vi "Category Manager GUI.vi"(8 "error in (no error)":errorcluster, 11 "Database.lvclass":refnum<class "Account History.lvclass">) -> (0 "error out":errorcluster, 3 "Database.lvclass":refnum<class "Account History.lvclass">)   [LabVIEW 2018]
uses:
  support/classes/database/Account History.lvclass
  <vilib>/Utility/miscctls.llb/LVRowAndColumnTypeDef.ctl
  support/classes/CategoryList/CategoryList.lvclass
panel:
  in  "Clear Amount":bool
  in  "Edit Amount":bool
  in  "Rename":bool
  in  "Delete":bool
  in  "Add":bool
  in  "Category Name":string
  in  "Category Table":i32(listbox)
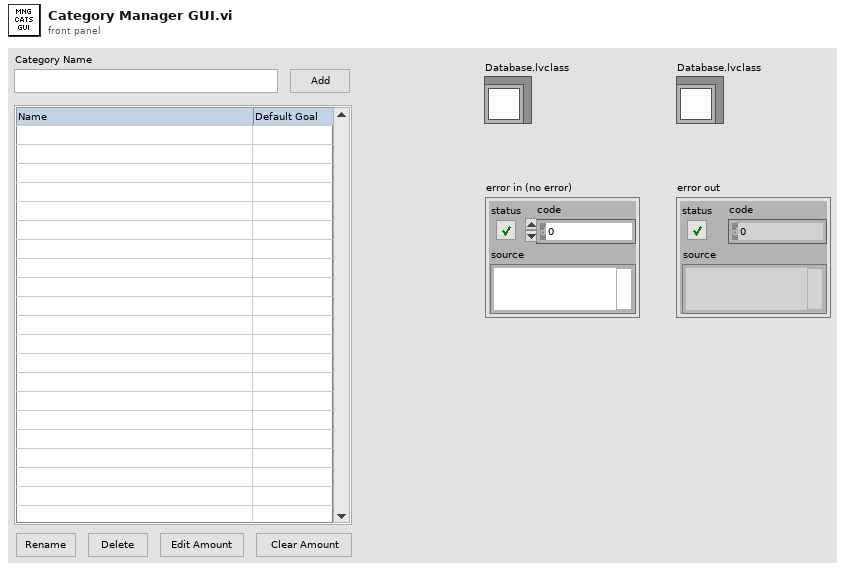
[diagram p1: front panel]
types:
  T1 = typedef "LVRowAndColumnTypeDef.ctl" = cluster{"Row":i32, "Column":i32}
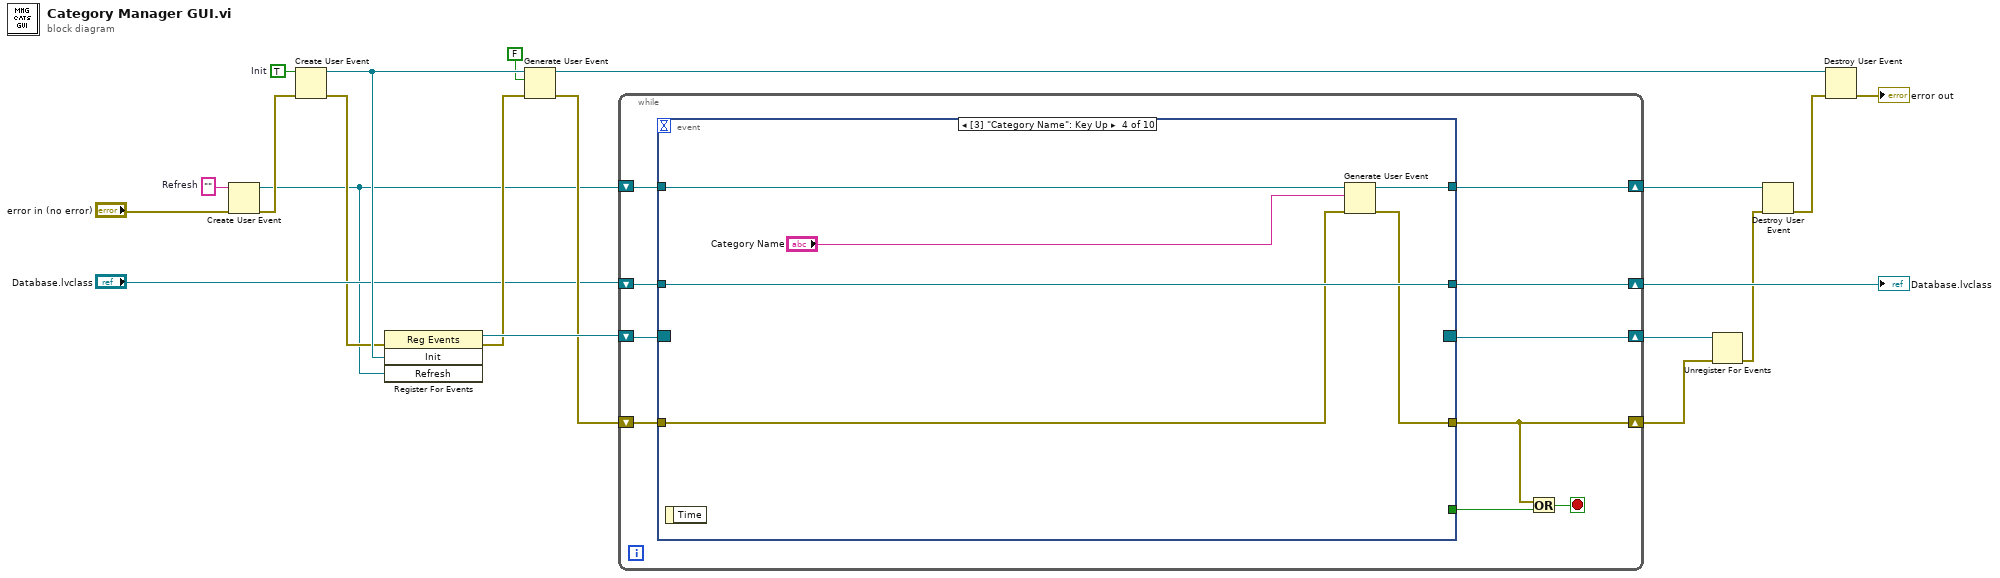
[diagram p0: block diagram]
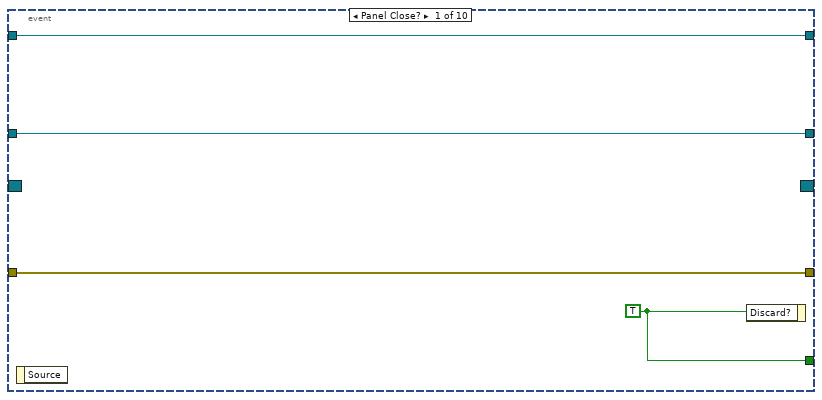
[diagram p2: hidden frame]
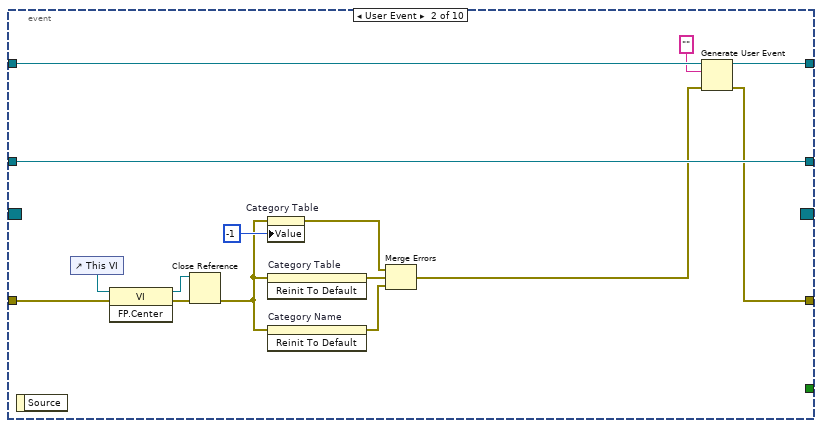
[diagram p3: hidden frame]
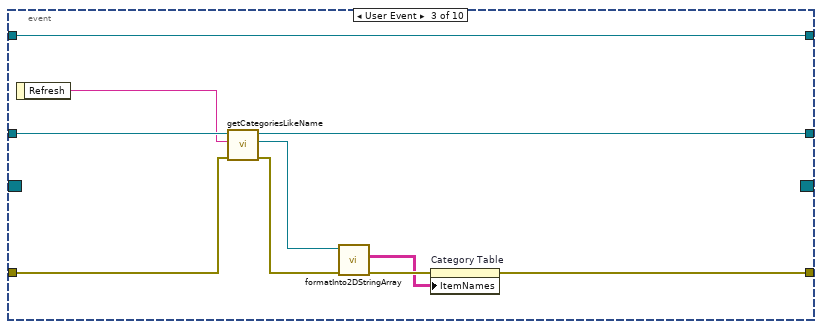
[diagram p4: hidden frame]
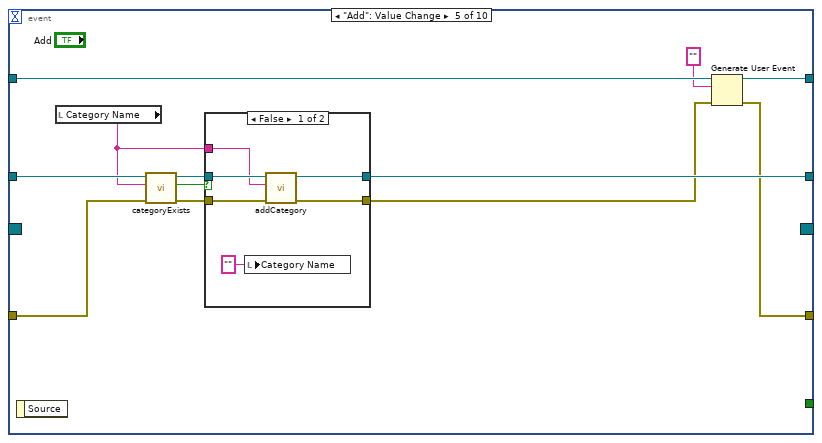
[diagram p5: hidden frame]
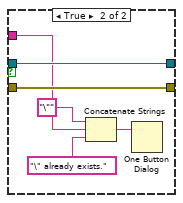
[diagram p6: hidden frame]
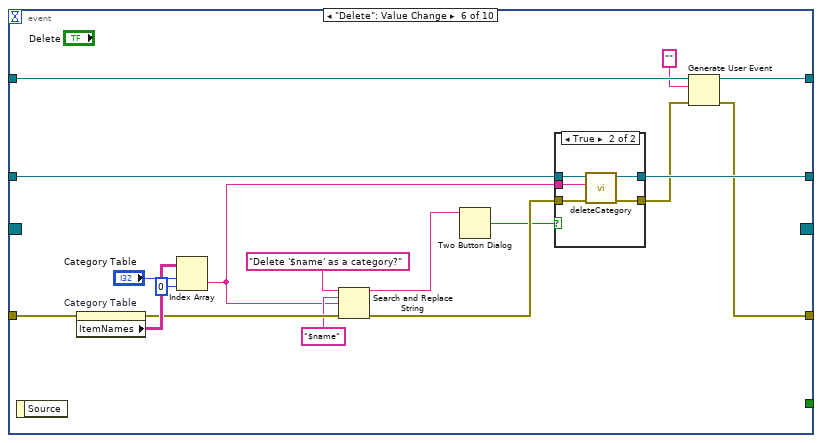
[diagram p7: hidden frame]
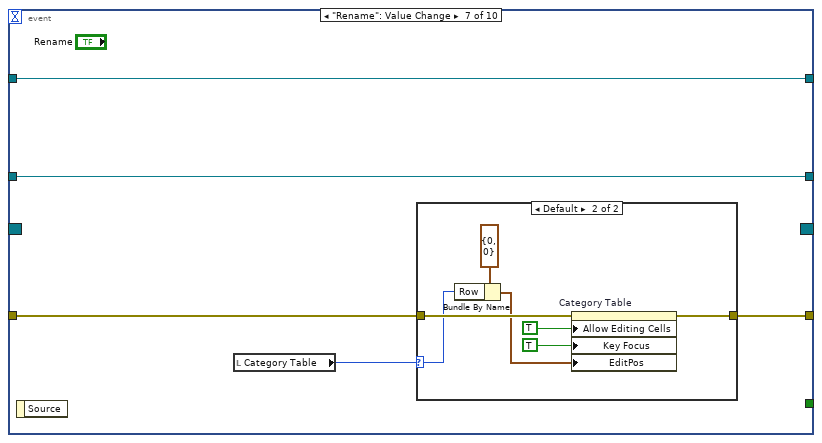
[diagram p9: hidden frame]
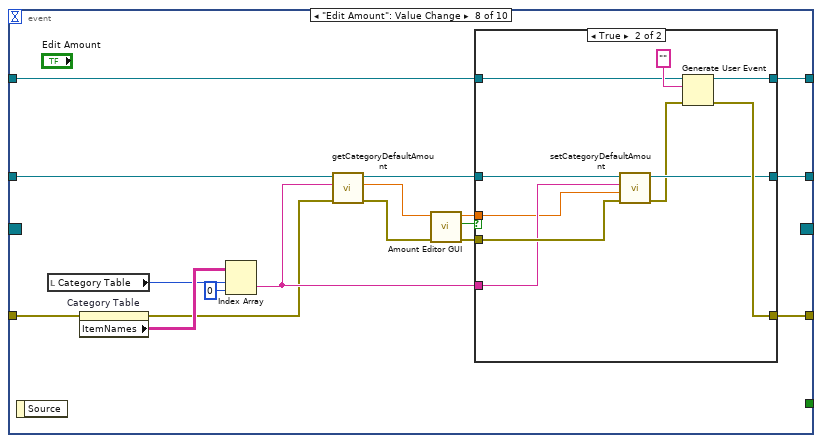
[diagram p11: hidden frame]
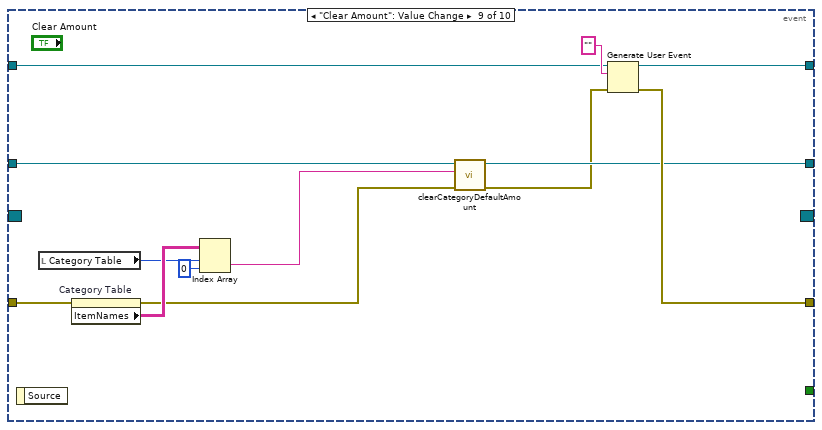
[diagram p13: hidden frame]
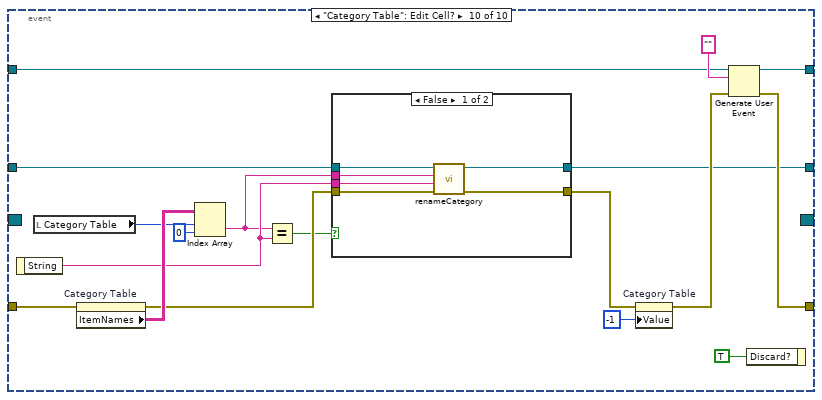
[diagram p14: hidden frame]
diagram:
  w1 = ""  # Refresh
  w20 = TRUE  # Init
  n1 = Create User Event(user event datatype=w1, error in="error in (no error)") -> (user event=w2:refnum<user-event>, error out=w4:errorcluster)
  n2 = Create User Event(user event datatype=w20, error in=w4) -> (user event=w18:refnum<user-event>, error out=w12:errorcluster)
  n3 = register-events(error in=w12, w18, w2) -> (reference out=w19:refnum<event-registration>, error out=w17:errorcluster)  [unwired: 1 in]
  n4 = Generate User Event(user event=w18, event data cluster=FALSE ("event data"), error in=w17) -> (user event out=w11:refnum<user-event>, error out=w16:errorcluster)  [unwired: 1 in]
  n5 = while {
    shift-right: [w28] -> w9
    shift-left: w19 -> [w30]
    shift-right: [w27] -> w8
    shift-left: w16 -> [w29]
    shift-right: [w23] -> w13
    shift-left: "Database.lvclass" -> [w24]
    shift-right: [w21] -> w5
    shift-left: w2 -> [w22]
    stop <- w25 stop-if-true
    n6 = event shown="[3] \"Category Name\": Key Up" {
      selector: w30 -> [_ _ _ _ _ _ _ _ _ _]
      dyn-events: [_ _ _ _ _ _ _ _ _ _] -> w28
      timeout: _ -> [_ _ _ _ _ _ _ _ _ _]
      tunnel: [w34 _ _ _ _ _ _ _ _ _] -> w26
      tunnel: w29 -> [w33 w45 w56 w61 w72 w107 w119 w138 w167 w186]
      tunnel: [w33 w36 w55 w62 w68 w100 w118 w142 w163 w180] -> w27
      tunnel: w24 -> [w32 w40 w58 w65 w74 w97 w116 w133 w162 w178]
      tunnel: [w32 w40 w57 w65 w71 w104 w116 w134 w161 w177] -> w23
      tunnel: w22 -> [w31 w39 w59 w64 w69 w102 w115 w143 w165 w181]
      tunnel: [w31 w38 w59 w63 w70 w103 w115 w144 w164 w182] -> w21
      event Panel Close? {
        w34 = TRUE ("Discard?")
        n7 = event-data() -> ()  [unwired: 1 in, 1 out]
        n8 = event-data("Discard?"=w34) -> ()  [unwired: 1 in, 1 out]
      }
      event User Event {
        n9 = event-data() -> ()  [unwired: 1 in, 1 out]
        n10 = control-ref of="This VI"() -> (w46:refnum<vi>)
        n11 = invoke class="VI" method="FP.Center"(reference=w46, error in=w45) -> (reference out=w43:refnum<vi>, error out=w44:errorcluster)  [unwired: 1 in, 1 out]
        n12 = Close Reference(reference=w43, error in (no error)=w44) -> (error out=w42:errorcluster)
        n13 = property on="Category Table" class="MCListbox (strict)"(error in=w42, "Value"=-1 ("Category Table")) -> (error out=w41:errorcluster)  [unwired: 1 in, 1 out]
        n14 = invoke on="Category Table" class="MCListbox (strict)" method="Reinit To Default"(error in=w42) -> (error out=w48:errorcluster)  [unwired: 2 in, 2 out]
        n15 = invoke on="Category Name" class="Str" method="Reinit To Default"(error in=w42) -> (error out=w49:errorcluster)  [unwired: 2 in, 2 out]
        n16 = Merge Errors(w41, w48, w49) -> (w37:errorcluster)
        n17 = Generate User Event(user event=w39, event data cluster="" ("event data"), error in=w37) -> (user event out=w38:refnum<user-event>, error out=w36:errorcluster)  [unwired: 1 in]
      }
      event User Event {
        n18 = event-data() -> ("Refresh"=w54:string)  [unwired: 1 in]
        n19 = call "getCategoriesLikeName.vi"("error in (no error)"=w56, "Name filter"=w54, "Database in"=w58) -> ("error out"=w52:errorcluster, "CategoryList out"=w53:refnum<class "CategoryList.lvclass">, "Database out"=w57:refnum<class "Account History.lvclass">)  [unwired: 6 in]
        n20 = call "formatInto2DStringArray.vi"("error in (no error)"=w52, "CategoryList in"=w53) -> ("error out"=w51:errorcluster, "2D String Array"=w50:string[][])  [unwired: 7 in, 1 out]
        n21 = property on="Category Table" class="MCListbox (strict)"(error in=w51, "ItemNames"=w50) -> (error out=w55:errorcluster)  [unwired: 1 in, 1 out]
      }
      event "Category Name": Key Up {
        n22 = event-data() -> ()  [unwired: 1 in, 1 out]
        n23 = Generate User Event(user event=w64, event data cluster="Category Name", error in=w61) -> (user event out=w63:refnum<user-event>, error out=w62:errorcluster)  [unwired: 1 in]
      }
      event "Add": Value Change {
        n24 = event-data() -> ()  [unwired: 1 in, 1 out]
        n25 = local read "Category Name"() -> (w73:string)
        n26 = call "categoryExists.vi"("error in (no error)"=w72, "Category Name"=w73, "Account History in"=w74) -> ("error out"=w76:errorcluster, "Exist?"=w77:bool, "Account History out"=w75:refnum<class "Account History.lvclass">)  [unwired: 6 in]
        n27 = case shown="False" w77 {
          tunnel: w76 -> [w82 w88]
          tunnel: w75 -> [w83 w89]
          tunnel: [w81 w89] -> w71
          tunnel: [w80 w88] -> w67
          tunnel: w73 -> [w79 w86]
          frame False {
            n28 = local write "Category Name"("" ("Category Name")) -> ()
            n29 = call "addCategory.vi"("error in (no error)"=w82, "name"=w79, "Database in"=w83) -> ("error out"=w80:errorcluster, "Database out"=w81:refnum<class "Account History.lvclass">)  [unwired: 7 in]
          }
          frame True {
            n30 = Concatenate Strings("\"" ("string"), w86, "\" already exists." ("string")) -> (w85:string)
            n31 = One Button Dialog(message=w85) -> ()  [unwired: 1 in, 1 out]
          }
        }
        n32 = Generate User Event(user event=w69, event data cluster="" ("Category Name"), error in=w67) -> (user event out=w70:refnum<user-event>, error out=w68:errorcluster)  [unwired: 1 in]
      }
      event "Delete": Value Change {
        n33 = event-data() -> ()  [unwired: 1 in, 1 out]
        n34 = property on="Category Table" class="MCListbox (strict)"(error in=w107) -> (error out=w96:errorcluster, "ItemNames"=w106:string[][])  [unwired: 1 in, 1 out]
        n35 = Index Array(array=w106, index (row)="Category Table", index (col)=0 ("disabled index (col)")) -> (element=w92:string)
        n36 = Search and Replace String(input string="Delete '$name' as a category?", search string="$name", replace string=w92, error in=w96) -> (result string=w91:string, error out=w95:errorcluster)  [unwired: 4 in, 2 out]
        n37 = Two Button Dialog(message=w91) -> (T button?=w90:bool)  [unwired: 2 in]
        n38 = case shown="True" w90 {
          tunnel: [w109 w114] -> w104
          tunnel: [w108 w113] -> w101
          tunnel: w97 -> [w109 w112]
          tunnel: w95 -> [w108 w111]
          tunnel: w92 -> [_ w110]
          frame False {
          }
          frame True {
            n39 = call "deleteCategory.vi"("error in (no error)"=w111, "Category Name"=w110, "Database in"=w112) -> ("error out"=w113:errorcluster, "Database out"=w114:refnum<class "Account History.lvclass">)  [unwired: 7 in]
          }
        }
        n40 = Generate User Event(user event=w102, event data cluster="" ("event data"), error in=w101) -> (user event out=w103:refnum<user-event>, error out=w100:errorcluster)  [unwired: 1 in]
      }
      event "Rename": Value Change {
        n41 = event-data() -> ()  [unwired: 1 in, 1 out]
        n42 = local read "Category Table"() -> (w117:i32)
        n43 = case shown="Default" w117 {
          selector: w117 -> [_ w121]
          tunnel: w119 -> [w120 w127]
          tunnel: [w120 w125] -> w118
          frame ..-1 {
          }
          frame Default {
            n44 = Bundle By Name(cluster=T1 {"Row"=0, "Column"=0} ("Edit Position"), "Row"=w121) -> (w122:T1)
            n45 = property on="Category Table" class="MCListbox (strict)"(error in=w127, "Allow Editing Cells"=TRUE, "Key Focus"=TRUE, "EditPos"=w122) -> (error out=w125:errorcluster)  [unwired: 1 in, 1 out]
          }
        }
      }
      event "Edit Amount": Value Change {
        n46 = event-data() -> ()  [unwired: 1 in, 1 out]
        n47 = local read "Category Table"() -> (w140:i32)
        n48 = property on="Category Table" class="MCListbox (strict)"(error in=w138) -> (error out=w130:errorcluster, "ItemNames"=w141:string[][])  [unwired: 1 in, 1 out]
        n49 = Index Array(array=w141, index (row)=w140, index (col)=0 ("disabled index (col)")) -> (element=w131:string)
        n50 = call "getCategoryDefaultAmount.vi"("error in (no error)"=w130, "Name"=w131, "Account History in"=w133) -> ("error out"=w129:errorcluster, "Default Amount"=w128:dbl, "Account History out"=w132:refnum<class "Account History.lvclass">)  [unwired: 6 in]
        n51 = call "Amount Editor GUI.vi"("error in (no error)"=w129, "Input Amount"=w128) -> ("error out"=w135:errorcluster, "UserConfirm?"=w136:bool, "Output Amount"=w137:dbl)  [unwired: 7 in]
        n52 = case shown="True" w136 {
          tunnel: [w147 w156] -> w144
          tunnel: w143 -> [w147 w155]
          tunnel: [w145 w154] -> w142
          tunnel: w137 -> [_ w148]
          tunnel: w135 -> [w145 w150]
          tunnel: w132 -> [w146 w153]
          tunnel: [w146 w152] -> w134
          tunnel: w131 -> [_ w149]
          frame False {
          }
          frame True {
            n53 = call "setCategoryDefaultAmount.vi"("error in (no error)"=w150, "Default Amount"=w148, "Name"=w149, "Account History in"=w153) -> ("error out"=w151:errorcluster, "Account History out"=w152:refnum<class "Account History.lvclass">)  [unwired: 6 in]
            n54 = Generate User Event(user event=w155, event data cluster="" ("event data"), error in=w151) -> (user event out=w156:refnum<user-event>, error out=w154:errorcluster)  [unwired: 1 in]
          }
        }
      }
      event "Clear Amount": Value Change {
        n55 = event-data() -> ()  [unwired: 1 in, 1 out]
        n56 = local read "Category Table"() -> (w169:i32)
        n57 = property on="Category Table" class="MCListbox (strict)"(error in=w167) -> (error out=w159:errorcluster, "ItemNames"=w170:string[][])  [unwired: 1 in, 1 out]
        n58 = Index Array(array=w170, index (row)=w169, index (col)=0 ("disabled index (col)")) -> (element=w158:string)
        n59 = call "clearCategoryDefaultAmount.vi"("error in (no error)"=w159, "Name"=w158, "Account History in"=w162) -> ("error out"=w160:errorcluster, "Account History out"=w161:refnum<class "Account History.lvclass">)  [unwired: 7 in]
        n60 = Generate User Event(user event=w165, event data cluster="" ("event data"), error in=w160) -> (user event out=w164:refnum<user-event>, error out=w163:errorcluster)  [unwired: 1 in]
      }
      event "Category Table": Edit Cell? {
        n61 = event-data() -> ("String"=w174:string)  [unwired: 1 in]
        n62 = local read "Category Table"() -> (w187:i32)
        n63 = property on="Category Table" class="MCListbox (strict)"(error in=w186) -> (error out=w175:errorcluster, "ItemNames"=w188:string[][])  [unwired: 1 in, 1 out]
        n64 = Index Array(array=w188, index (row)=w187, index (col)=0 ("disabled index (col)")) -> (element=w171:string)
        n65 = Equal?(x=w171, y=w174) -> (x = y?=w173:bool)
        n66 = case shown="False" w173 {
          tunnel: w178 -> [w190 w196]
          tunnel: [w194 w196] -> w177
          tunnel: [w193 w195] -> w176
          tunnel: w175 -> [w189 w195]
          tunnel: w171 -> [w191 _]
          tunnel: w174 -> [w192 _]
          frame False {
            n67 = call "renameCategory.vi"("error in (no error)"=w189, "New Name"=w192, "Current Name"=w191, "Database in"=w190) -> ("error out"=w193:errorcluster, "Database out"=w194:refnum<class "Account History.lvclass">)  [unwired: 6 in]
          }
          frame True {
          }
        }
        n68 = property on="Category Table" class="MCListbox (strict)"(error in=w176, "Value"=-1 ("Category Table")) -> (error out=w179:errorcluster)  [unwired: 1 in, 1 out]
        n69 = Generate User Event(user event=w181, event data cluster="", error in=w179) -> (user event out=w182:refnum<user-event>, error out=w180:errorcluster)  [unwired: 1 in]
        n70 = event-data("Discard?"=TRUE) -> ()  [unwired: 1 in, 1 out]
      }
    }
    n71 = Or(x=w27, y=w26) -> (x .or. y?=w25:bool)
  }
  "Database.lvclass" <- w13
  n72 = Unregister For Events(event registration refnum=w9, error in=w8) -> (error out=w10:errorcluster)
  n73 = Destroy User Event(user event=w5, error in=w10) -> (error out=w7:errorcluster)
  n74 = Destroy User Event(user event=w11, error in=w7) -> (error out=→"error out":errorcluster)
